vi "Class_Find Match Indexes.vi"(4 "Groups to Find":refnum<class>[](array[class]), 5 "GroupList":refnum<class>[](array[class])) -> (1 "Indexes":i32[](array[numeric]))   [LabVIEW 2015]
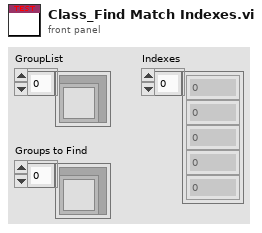
[diagram p1: front panel]
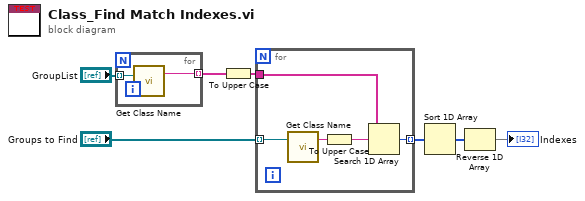
[diagram p0: block diagram]
diagram:
  n1 = for {
    tunnel: "GroupList" -> [w9] mode=indexing
    tunnel: [w8] -> w3 mode=indexing
    n2 = call "Get Class Name.vi"("lvclass"=w9) -> ("Child Name"=w8:string)  [unwired: 3 in, 1 out]
  }
  n3 = To Upper Case(1:w3) -> (0:w2:string[])
  n4 = for {
    tunnel: "Groups to Find" -> [w14] mode=indexing
    tunnel: w2 -> [w11]
    tunnel: [w10] -> w4 mode=indexing
    n5 = call "Get Class Name.vi"("lvclass"=w14) -> ("Child Name"=w13:string)  [unwired: 3 in, 1 out]
    n6 = To Upper Case(1:w13) -> (0:w12:string)
    n7 = Search 1D Array(1D array=w11, element=w12) -> (index of element=w10:i32)  [unwired: 1 in]
  }
  n8 = Sort 1D Array(array=w4) -> (sorted array=w5:i32[])
  n9 = Reverse 1D Array(array=w5) -> (reversed array=→"Indexes":i32[])
